vi "Evaluate Value Change Trigger.vi"(8 "error in (no error)":errorcluster, 10 "Trigger Data":dbl[](array[numeric]), 11 "Value Change Trigger in":refnum<class "Value Change Trigger.lvclass">) -> (0 "error out":errorcluster, 2 "Trigger":bool, 3 "Value Change Trigger out":refnum<class "Value Change Trigger.lvclass">)   [LabVIEW 2015, in "Value Change Trigger.lvclass"]
uses:
  Value Change Trigger.lvclass
  Value Change Trigger.lvclass/Value Change Trigger.ctl
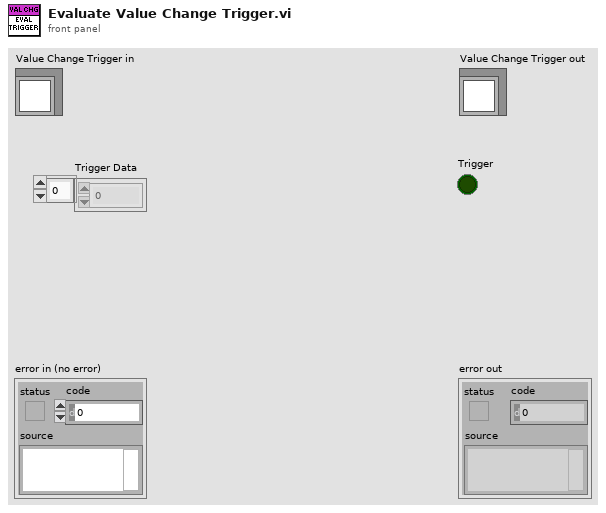
[diagram p1: front panel]
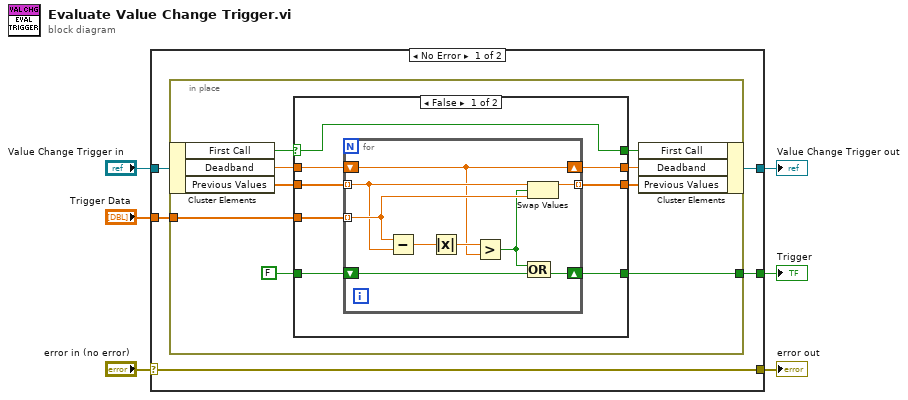
[diagram p0: block diagram]
diagram:
  n1 = case shown="No Error" "error in (no error)" {
    selector: "error in (no error)" -> [w7 w41]
    tunnel: "Value Change Trigger in" -> [w11 w42]
    tunnel: [w10 w42] -> w5
    tunnel: "Trigger Data" -> [w9 _]
    tunnel: [w8 _] -> w3
    tunnel: [w7 w41] -> w1
    frame No Error {
      n2 = in-place {
        in-place-border: w9 -> [w14]
        in-place-border: [w17] -> w8
        n3 = in-place-cluster #1(w11) -> ("First Call"=w20:bool, "Deadband"=w15:dbl, "Previous Values"=w19:dbl[])
        n4 = case shown="False" w20 {
          selector: w20 -> [w22 _]
          tunnel: w19 -> [w26 _]
          tunnel: [w27 w39] -> w18
          tunnel: w14 -> [w28 w39]
          tunnel: [w25 w38] -> w17
          tunnel: [w23 w40] -> w16
          tunnel: w15 -> [w24 w40]
          tunnel: [w22 _] -> w13
          tunnel: FALSE -> [w21 w38]
          frame False {
            n5 = for {
              tunnel: w28 -> [w35] mode=indexing
              tunnel: [w34] -> w27 mode=indexing
              tunnel: w26 -> [w33] mode=indexing
              shift-right: [w30] -> w25
              shift-left: w21 -> [w31]
              shift-right: [w29] -> w23
              shift-left: w24 -> [w29]
              n6 = Subtract(x=w35, y=w33) -> (x-y=w36:dbl)
              n7 = Absolute Value(x=w36) -> (abs(x)=w37:dbl)
              n8 = Greater?(x=w37, y=w29) -> (0:w32:bool)
              n9 = Swap Values(12:w33, 13:w32, 14:w35) -> (1:w34:dbl)  [unwired: 1 out]
              n10 = Compound Arithmetic op=OR(w32, w31) -> (w30:bool)
            }
          }
          frame True {
            # "Just latch the trigger channel values on first call."
          }
        }
        n11 = in-place-cluster #1("First Call"=w13, "Deadband"=w16, "Previous Values"=w18) -> (w10:refnum<class "Value Change Trigger.lvclass">)
      }
    }
    frame Error {
    }
  }
  "error out" <- w1
  "Value Change Trigger out" <- w5
  "Trigger" <- w3
